vi "Process_Oculus_Data - Rachel.vi"(5 "Arm X Min":dbl, 7 "Arm X Max":dbl, 8 "error in":errorcluster, 9 "Calibration Data in":T3, 10 "Control in":enum16{"Calibrate", "Max", "Min"}(ring), 11 "Oculus Data In":T2) -> (0 "error out":errorcluster, 1 "Calibration Data out":T3, 3 "Oculus Data out":T1)   [LabVIEW 2017]
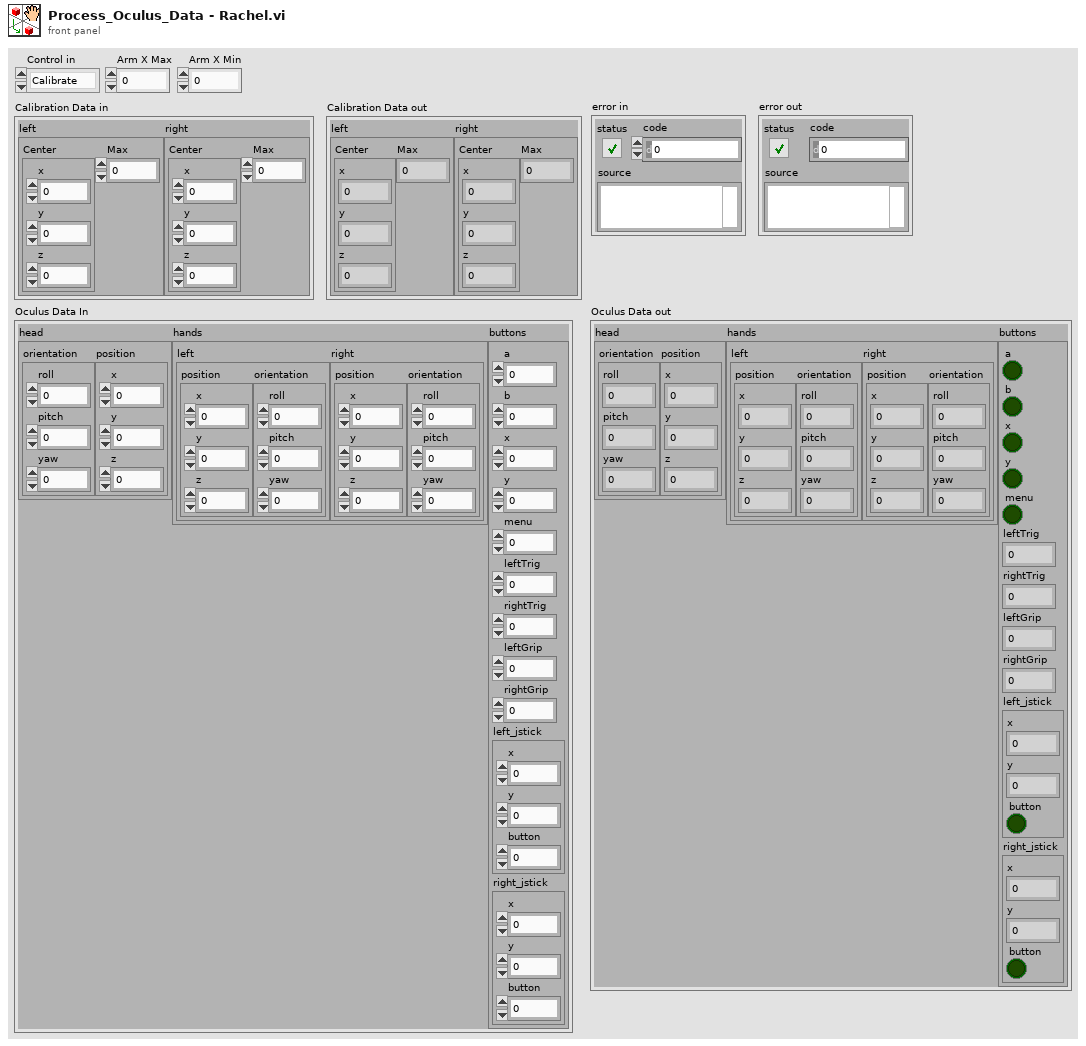
[diagram p1: front panel]
types:
  T1 = cluster{"head":cluster{"orientation":cluster{"roll":dbl, "pitch":dbl, "yaw":dbl}, "position":cluster{"x":dbl, "y":dbl, "z":dbl}}, "hands":cluster{"left":cluster{"position":cluster{"x":dbl, "y":dbl, "z":dbl}, "orientation":cluster{"roll":dbl, "pitch":dbl, "yaw":dbl}}, "right":cluster{"position":cluster{"x":dbl, "y":dbl, "z":dbl}, "orientation":cluster{"roll":dbl, "pitch":dbl, "yaw":dbl}}}, "buttons":cluster{"a":bool, "b":bool, "x":bool, "y":bool, "menu":bool, "leftTrig":dbl, "rightTrig":dbl, "leftGrip":dbl, "rightGrip":dbl, "left_jstick":cluster{"x":dbl, "y":dbl, "button":bool}, "right_jstick":cluster{"x":dbl, "y":dbl, "button":bool}}}
  T2 = cluster{"head":cluster{"orientation":cluster{"roll":dbl, "pitch":dbl, "yaw":dbl}, "position":cluster{"x":dbl, "y":dbl, "z":dbl}}, "hands":cluster{"left":cluster{"position":cluster{"x":dbl, "y":dbl, "z":dbl}, "orientation":cluster{"roll":dbl, "pitch":dbl, "yaw":dbl}}, "right":cluster{"position":cluster{"x":dbl, "y":dbl, "z":dbl}, "orientation":cluster{"roll":dbl, "pitch":dbl, "yaw":dbl}}}, "buttons":cluster{"a":i32, "b":i32, "x":i32, "y":i32, "menu":i32, "leftTrig":dbl, "rightTrig":dbl, "leftGrip":dbl, "rightGrip":dbl, "left_jstick":cluster{"x":dbl, "y":dbl, "button":i32}, "right_jstick":cluster{"x":dbl, "y":dbl, "button":i32}}}
  T3 = cluster{"left":cluster{"Center":cluster{"x":dbl, "y":dbl, "z":dbl}, "Max":dbl}, "right":cluster{"Center":cluster{"x":dbl, "y":dbl, "z":dbl}, "Max":dbl}}
  T4 = cluster{"orientation":cluster{"roll":dbl, "pitch":dbl, "yaw":dbl}, "position":cluster{"x":dbl, "y":dbl, "z":dbl}}
  T5 = cluster{"left":cluster{"position":cluster{"x":dbl, "y":dbl, "z":dbl}, "orientation":cluster{"roll":dbl, "pitch":dbl, "yaw":dbl}}, "right":cluster{"position":cluster{"x":dbl, "y":dbl, "z":dbl}, "orientation":cluster{"roll":dbl, "pitch":dbl, "yaw":dbl}}}
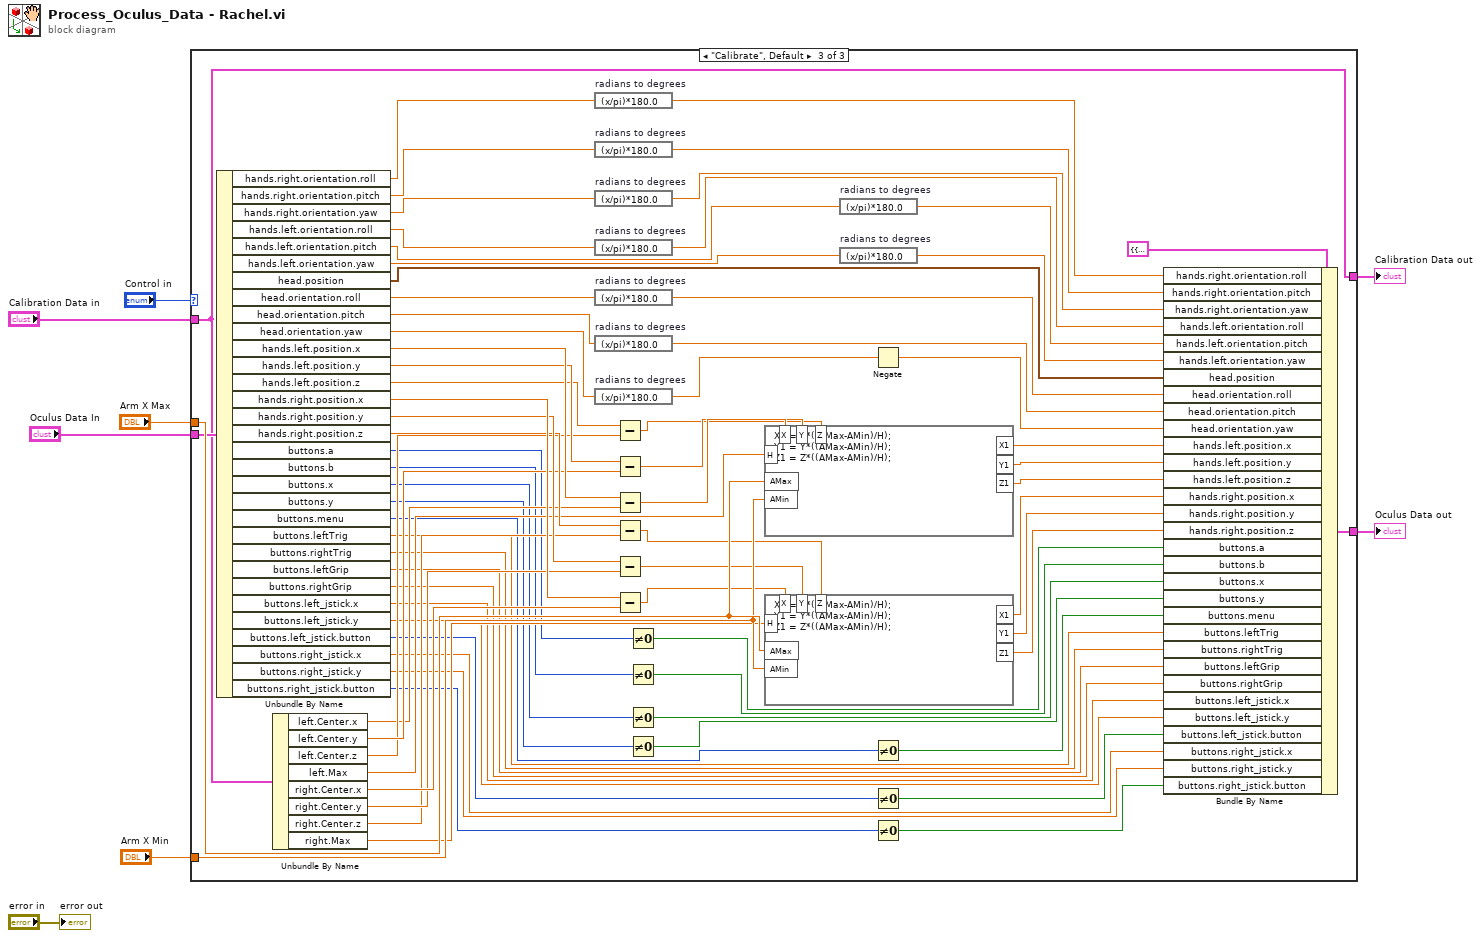
[diagram p0: block diagram]
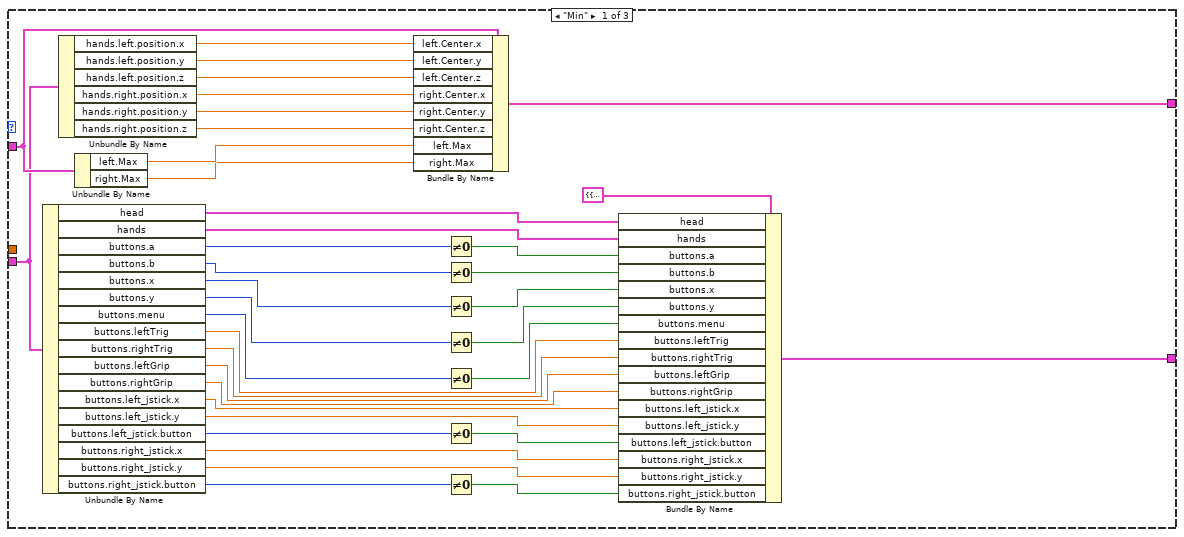
[diagram p2: hidden frame]
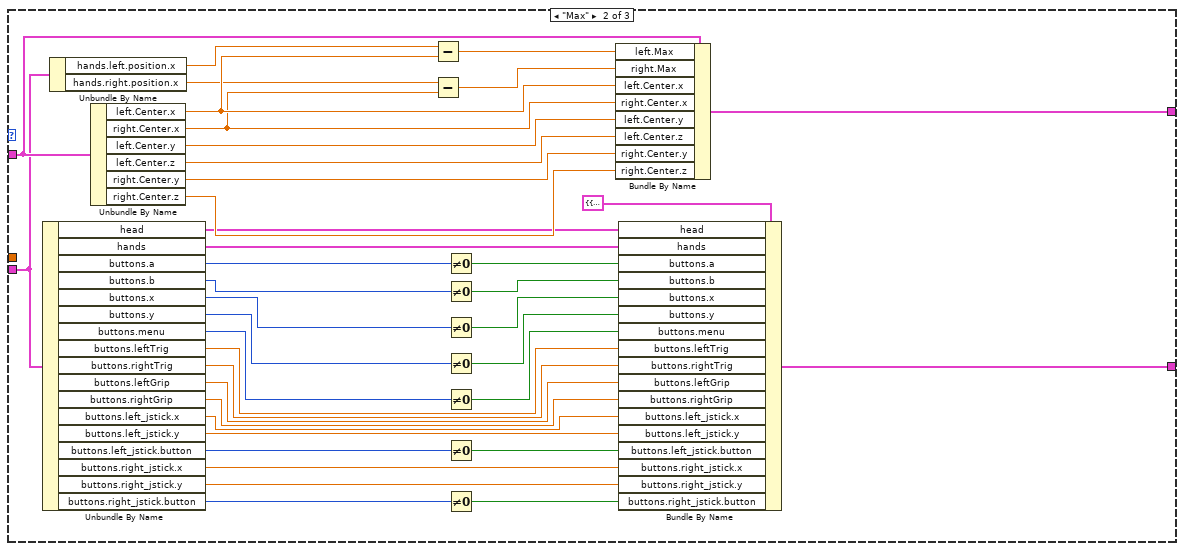
[diagram p3: hidden frame]
diagram:
  n1 = case shown="\"Calibrate\", Default" "Control in" {
    tunnel: "Oculus Data In" -> [w9 w72 w146]
    tunnel: "Arm X Max" -> [_ _ w154]
    tunnel: "Arm X Min" -> [_ _ w153]
    tunnel: "Calibration Data in" -> [w45 w75 w129]
    tunnel: [w42 w84 w129] -> w4
    tunnel: [w10 w68 w98] -> w2
    frame "Min" {
      n2 = Unbundle By Name(w9) -> ("head"=w34:T4, "hands"=w33:T5, "buttons.a"=w32:i32, "buttons.b"=w31:i32, "buttons.x"=w30:i32, "buttons.y"=w29:i32, "buttons.menu"=w24:i32, "buttons.leftTrig"=w18:dbl, "buttons.rightTrig"=w17:dbl, "buttons.leftGrip"=w16:dbl, "buttons.rightGrip"=w15:dbl, "buttons.left_jstick.x"=w14:dbl, "buttons.left_jstick.y"=w13:dbl, "buttons.left_jstick.button"=w22:i32, "buttons.right_jstick.x"=w12:dbl, "buttons.right_jstick.y"=w11:dbl, "buttons.right_jstick.button"=w21:i32)
      n3 = Unbundle By Name(w9) -> ("hands.left.position.x"=w41:dbl, "hands.left.position.y"=w40:dbl, "hands.left.position.z"=w39:dbl, "hands.right.position.x"=w38:dbl, "hands.right.position.y"=w37:dbl, "hands.right.position.z"=w36:dbl)
      n4 = Unbundle By Name(w45) -> ("left.Max"=w44:dbl, "right.Max"=w43:dbl)
      n5 = Bundle By Name(cluster=w45, "left.Center.x"=w41, "left.Center.y"=w40, "left.Center.z"=w39, "right.Center.x"=w38, "right.Center.y"=w37, "right.Center.z"=w36, "left.Max"=w44, "right.Max"=w43) -> (w42:T3)
      n6 = Not Equal To 0?(x=w32) -> (x != 0?=w28:bool)
      n7 = Not Equal To 0?(x=w31) -> (x != 0?=w27:bool)
      n8 = Not Equal To 0?(x=w30) -> (x != 0?=w26:bool)
      n9 = Not Equal To 0?(x=w29) -> (x != 0?=w25:bool)
      n10 = Not Equal To 0?(x=w24) -> (x != 0?=w23:bool)
      n11 = Not Equal To 0?(x=w22) -> (x != 0?=w20:bool)
      n12 = Not Equal To 0?(x=w21) -> (x != 0?=w19:bool)
      n13 = Bundle By Name(cluster=T1 {"head"={"orientation"={"roll"=0.0, "pitch"=0.0, "yaw"=0.0}, "position"={"x"=0.0, "y"=0.0, "z"=0.0}}, "hands"={"left"={"position"={"x"=0.0, "y"=0.0, "z"=0.0}, "orientation"={"roll"=0.0, "pitch"=0.0, "yaw"=0.0}}, "right"={"position"={"x"=0.0, "y"=0.0, "z"=0.0}, "orientation"={"roll"=0.0, "pitch"=0.0, "yaw"=0.0}}}, "buttons"={"a"=FALSE, "b"=FALSE, "x"=FALSE, "y"=FALSE, "menu"=FALSE, "leftTrig"=0.0, "rightTrig"=0.0, "leftGrip"=0.0, "rightGrip"=0.0, "left_jstick"={"x"=0.0, "y"=0.0, "button"=FALSE}, "right_jstick"={"x"=0.0, "y"=0.0, "button"=FALSE}}} ("Oculus Data out"), "head"=w34, "hands"=w33, "buttons.a"=w28, "buttons.b"=w27, "buttons.x"=w26, "buttons.y"=w25, "buttons.menu"=w23, "buttons.leftTrig"=w18, "buttons.rightTrig"=w17, "buttons.leftGrip"=w16, "buttons.rightGrip"=w15, "buttons.left_jstick.x"=w14, "buttons.left_jstick.y"=w13, "buttons.left_jstick.button"=w20, "buttons.right_jstick.x"=w12, "buttons.right_jstick.y"=w11, "buttons.right_jstick.button"=w19) -> (w10:T1)
    }
    frame "Max" {
      n14 = Unbundle By Name(w72) -> ("head"=w70:T4, "hands"=w69:T5, "buttons.a"=w67:i32, "buttons.b"=w66:i32, "buttons.x"=w65:i32, "buttons.y"=w64:i32, "buttons.menu"=w59:i32, "buttons.leftTrig"=w53:dbl, "buttons.rightTrig"=w52:dbl, "buttons.leftGrip"=w51:dbl, "buttons.rightGrip"=w50:dbl, "buttons.left_jstick.x"=w49:dbl, "buttons.left_jstick.y"=w48:dbl, "buttons.left_jstick.button"=w57:i32, "buttons.right_jstick.x"=w47:dbl, "buttons.right_jstick.y"=w46:dbl, "buttons.right_jstick.button"=w56:i32)
      n15 = Unbundle By Name(w72) -> ("hands.left.position.x"=w74:dbl, "hands.right.position.x"=w73:dbl)
      n16 = Unbundle By Name(w75) -> ("left.Center.x"=w83:dbl, "right.Center.x"=w82:dbl, "left.Center.y"=w81:dbl, "left.Center.z"=w80:dbl, "right.Center.y"=w79:dbl, "right.Center.z"=w78:dbl)
      n17 = Subtract(x=w74, y=w83) -> (x-y=w77:dbl)
      n18 = Subtract(x=w73, y=w82) -> (x-y=w76:dbl)
      n19 = Not Equal To 0?(x=w67) -> (x != 0?=w63:bool)
      n20 = Not Equal To 0?(x=w66) -> (x != 0?=w62:bool)
      n21 = Not Equal To 0?(x=w65) -> (x != 0?=w61:bool)
      n22 = Not Equal To 0?(x=w64) -> (x != 0?=w60:bool)
      n23 = Not Equal To 0?(x=w59) -> (x != 0?=w58:bool)
      n24 = Not Equal To 0?(x=w57) -> (x != 0?=w55:bool)
      n25 = Not Equal To 0?(x=w56) -> (x != 0?=w54:bool)
      n26 = Bundle By Name(cluster=w75, "left.Max"=w77, "right.Max"=w76, "left.Center.x"=w83, "right.Center.x"=w82, "left.Center.y"=w81, "left.Center.z"=w80, "right.Center.y"=w79, "right.Center.z"=w78) -> (w84:T3)
      n27 = Bundle By Name(cluster=T1 {"head"={"orientation"={"roll"=0.0, "pitch"=0.0, "yaw"=0.0}, "position"={"x"=0.0, "y"=0.0, "z"=0.0}}, "hands"={"left"={"position"={"x"=0.0, "y"=0.0, "z"=0.0}, "orientation"={"roll"=0.0, "pitch"=0.0, "yaw"=0.0}}, "right"={"position"={"x"=0.0, "y"=0.0, "z"=0.0}, "orientation"={"roll"=0.0, "pitch"=0.0, "yaw"=0.0}}}, "buttons"={"a"=FALSE, "b"=FALSE, "x"=FALSE, "y"=FALSE, "menu"=FALSE, "leftTrig"=0.0, "rightTrig"=0.0, "leftGrip"=0.0, "rightGrip"=0.0, "left_jstick"={"x"=0.0, "y"=0.0, "button"=FALSE}, "right_jstick"={"x"=0.0, "y"=0.0, "button"=FALSE}}} ("Oculus Data out"), "head"=w70, "hands"=w69, "buttons.a"=w63, "buttons.b"=w62, "buttons.x"=w61, "buttons.y"=w60, "buttons.menu"=w58, "buttons.leftTrig"=w53, "buttons.rightTrig"=w52, "buttons.leftGrip"=w51, "buttons.rightGrip"=w50, "buttons.left_jstick.x"=w49, "buttons.left_jstick.y"=w48, "buttons.left_jstick.button"=w55, "buttons.right_jstick.x"=w47, "buttons.right_jstick.y"=w46, "buttons.right_jstick.button"=w54) -> (w68:T1)
    }
    frame "Calibrate", Default {
      n28 = Unbundle By Name(w146) -> ("hands.right.orientation.roll"=w110:dbl, "hands.right.orientation.pitch"=w109:dbl, "hands.right.orientation.yaw"=w108:dbl, "hands.left.orientation.roll"=w104:dbl, "hands.left.orientation.pitch"=w103:dbl, "hands.left.orientation.yaw"=w102:dbl, "head.position"=w145:cluster{"x":dbl, "y":dbl, "z":dbl}, "head.orientation.roll"=w149:dbl, "head.orientation.pitch"=w148:dbl, "head.orientation.yaw"=w147:dbl, "hands.left.position.x"=w138:dbl, "hands.left.position.y"=w137:dbl, "hands.left.position.z"=w136:dbl, "hands.right.position.x"=w135:dbl, "hands.right.position.y"=w134:dbl, "hands.right.position.z"=w133:dbl, "buttons.a"=w120:i32, "buttons.b"=w114:i32, "buttons.x"=w118:i32, "buttons.y"=w115:i32, "buttons.menu"=w96:i32, "buttons.leftTrig"=w112:dbl, "buttons.rightTrig"=w111:dbl, "buttons.leftGrip"=w86:dbl, "buttons.rightGrip"=w85:dbl, "buttons.left_jstick.x"=w94:dbl, "buttons.left_jstick.y"=w93:dbl, "buttons.left_jstick.button"=w92:i32, "buttons.right_jstick.x"=w90:dbl, "buttons.right_jstick.y"=w89:dbl, "buttons.right_jstick.button"=w88:i32)
      n29 = Unbundle By Name(w129) -> ("left.Center.x"=w126:dbl, "left.Center.y"=w128:dbl, "left.Center.z"=w127:dbl, "left.Max"=w125:dbl, "right.Center.x"=w124:dbl, "right.Center.y"=w123:dbl, "right.Center.z"=w122:dbl, "right.Max"=w121:dbl)
      n30 = expression code="(x/pi)*180.0" "radians to degrees"(w110) -> (w107:dbl)
      n31 = expression code="(x/pi)*180.0" "radians to degrees"(w109) -> (w106:dbl)
      n32 = expression code="(x/pi)*180.0" "radians to degrees"(w108) -> (w105:dbl)
      n33 = expression code="(x/pi)*180.0" "radians to degrees"(w104) -> (w101:dbl)
      n34 = expression code="(x/pi)*180.0" "radians to degrees"(w149) -> (w144:dbl)
      n35 = expression code="(x/pi)*180.0" "radians to degrees"(w148) -> (w143:dbl)
      n36 = expression code="(x/pi)*180.0" "radians to degrees"(w147) -> (w158:dbl)
      n37 = Subtract(x=w136, y=w127) -> (x-y=w155:dbl)
      n38 = Subtract(x=w137, y=w128) -> (x-y=w156:dbl)
      n39 = Subtract(x=w138, y=w126) -> (x-y=w157:dbl)
      n40 = Subtract(x=w133, y=w122) -> (x-y=w150:dbl)
      n41 = Subtract(x=w134, y=w123) -> (x-y=w151:dbl)
      n42 = Subtract(x=w135, y=w124) -> (x-y=w152:dbl)
      n43 = Not Equal To 0?(x=w120) -> (x != 0?=w119:bool)
      n44 = Not Equal To 0?(x=w114) -> (x != 0?=w113:bool)
      n45 = Not Equal To 0?(x=w118) -> (x != 0?=w117:bool)
      n46 = Not Equal To 0?(x=w115) -> (x != 0?=w116:bool)
      n47 = formula code="X1 = X*((AMax-AMin)/H);\nY1 = Y*((AMax-AMin)/H);\nZ1 = Z*((AMax-AMin)/H);"("H"=w125, "AMax"=w154, "X"=w157, "Y"=w156, "Z"=w155, "AMin"=w153) -> ("X1"=w141:dbl, "Y1"=w140:dbl, "Z1"=w139:dbl)
      n48 = formula code="X1 = X*((AMax-AMin)/H);\nY1 = Y*((AMax-AMin)/H);\nZ1 = Z*((AMax-AMin)/H);"("H"=w121, "AMax"=w154, "X"=w152, "Y"=w151, "Z"=w150, "AMin"=w153) -> ("X1"=w132:dbl, "Y1"=w131:dbl, "Z1"=w130:dbl)
      n49 = expression code="(x/pi)*180.0" "radians to degrees"(w103) -> (w100:dbl)
      n50 = expression code="(x/pi)*180.0" "radians to degrees"(w102) -> (w99:dbl)
      n51 = Negate(x=w158) -> (-x=w142:dbl)
      n52 = Not Equal To 0?(x=w96) -> (x != 0?=w95:bool)
      n53 = Not Equal To 0?(x=w92) -> (x != 0?=w91:bool)
      n54 = Not Equal To 0?(x=w88) -> (x != 0?=w87:bool)
      n55 = Bundle By Name(cluster=T1 {"head"={"orientation"={"roll"=0.0, "pitch"=0.0, "yaw"=0.0}, "position"={"x"=0.0, "y"=0.0, "z"=0.0}}, "hands"={"left"={"position"={"x"=0.0, "y"=0.0, "z"=0.0}, "orientation"={"roll"=0.0, "pitch"=0.0, "yaw"=0.0}}, "right"={"position"={"x"=0.0, "y"=0.0, "z"=0.0}, "orientation"={"roll"=0.0, "pitch"=0.0, "yaw"=0.0}}}, "buttons"={"a"=FALSE, "b"=FALSE, "x"=FALSE, "y"=FALSE, "menu"=FALSE, "leftTrig"=0.0, "rightTrig"=0.0, "leftGrip"=0.0, "rightGrip"=0.0, "left_jstick"={"x"=0.0, "y"=0.0, "button"=FALSE}, "right_jstick"={"x"=0.0, "y"=0.0, "button"=FALSE}}} ("Oculus Data out"), "hands.right.orientation.roll"=w107, "hands.right.orientation.pitch"=w106, "hands.right.orientation.yaw"=w105, "hands.left.orientation.roll"=w101, "hands.left.orientation.pitch"=w100, "hands.left.orientation.yaw"=w99, "head.position"=w145, "head.orientation.roll"=w144, "head.orientation.pitch"=w143, "head.orientation.yaw"=w142, "hands.left.position.x"=w141, "hands.left.position.y"=w140, "hands.left.position.z"=w139, "hands.right.position.x"=w132, "hands.right.position.y"=w131, "hands.right.position.z"=w130, "buttons.a"=w119, "buttons.b"=w113, "buttons.x"=w117, "buttons.y"=w116, "buttons.menu"=w95, "buttons.leftTrig"=w112, "buttons.rightTrig"=w111, "buttons.leftGrip"=w86, "buttons.rightGrip"=w85, "buttons.left_jstick.x"=w94, "buttons.left_jstick.y"=w93, "buttons.left_jstick.button"=w91, "buttons.right_jstick.x"=w90, "buttons.right_jstick.y"=w89, "buttons.right_jstick.button"=w87) -> (w98:T1)
    }
  }
  "Calibration Data out" <- w4
  "Oculus Data out" <- w2
  "error out" <- "error in"
